vi "GSP_Manager_Wavelength_driver.vi"(4 "error in (no error)":errorcluster, 6 "Target (Move Only)":T1 {"Move type" items=["Both", "Grating Only", "Camera Only"]}, 7 "Action":T3) -> (0 "error out":errorcluster, 2 "VI reference (launch only)":refnum<vi>)   [LabVIEW 2015]
doc: "Provides an interface to the Camera Stage Manager. See the actions below.\n\nLaunch - launch the manager thread supplying references to the controls that the thread will update.\n\nHome - Home the camera stage\n\nMove - Move the camera to the position supplied by Target (in degrees)\n\nShutdown - Shutdown the camera stage manager"
uses:
  wavelength_driver_actions.ctl
  wavelength_parameters.ctl
  movetypes.ctl
  SystemUtil/Command.ctl
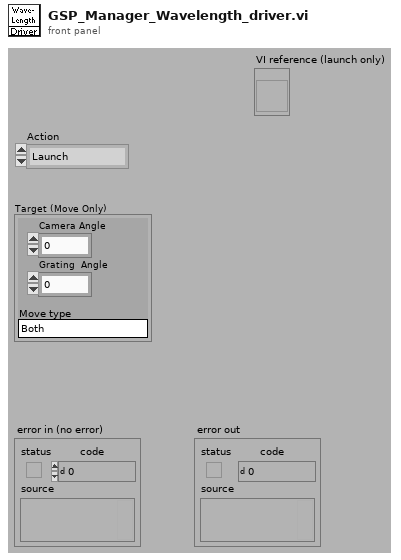
[diagram p1: front panel]
types:
  T1 = typedef "wavelength_parameters.ctl" = cluster{"Camera Angle":dbl, "Grating  Angle":dbl, "Move type":T2}
  T2 = typedef "movetypes.ctl" = u16
  T3 = typedef "wavelength_driver_actions.ctl" = enum16{"Launch", "Flexure On", "Flexure Off", "Move", "Home", "Shutdown"}
  T4 = typedef "Command.ctl" = cluster{"Command":string, "Parameter":string}
  T5 = cluster{string, "type string":i16[], "data string":string}
  T6 = cluster{string, "type string":i16[], "data string":string}[]
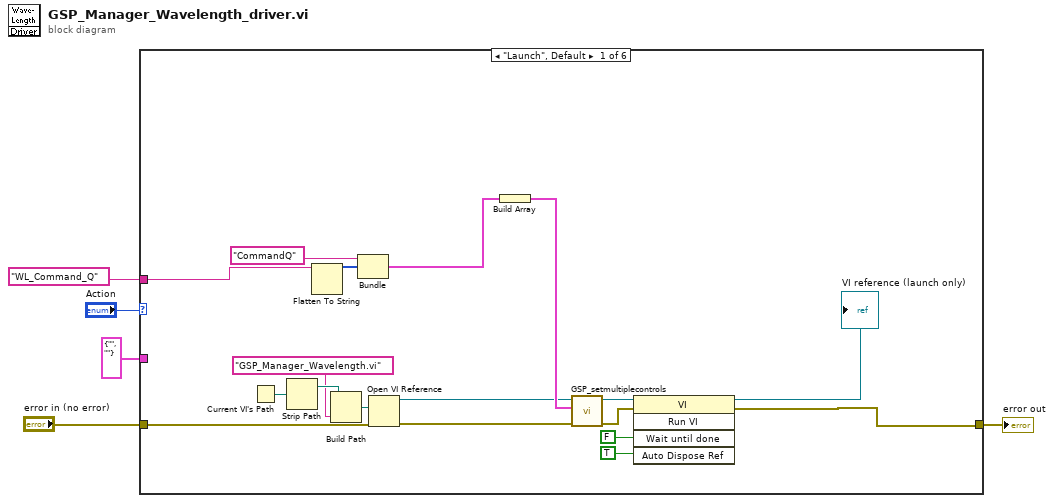
[diagram p0: block diagram]
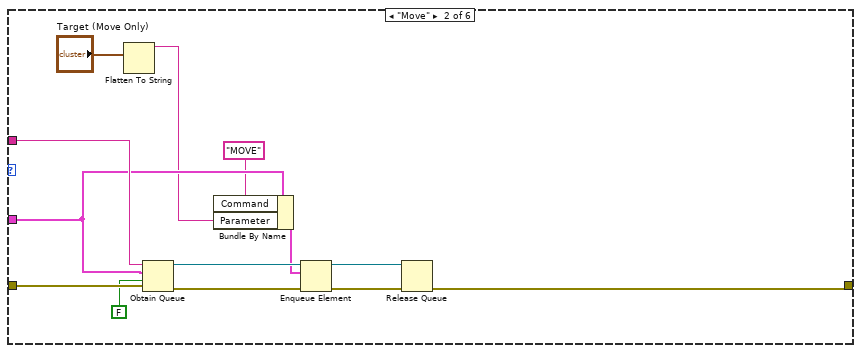
[diagram p2: hidden frame]
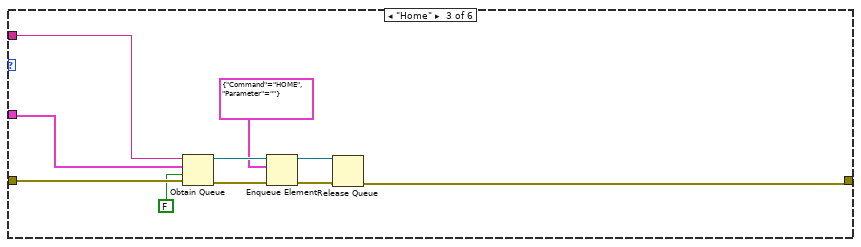
[diagram p3: hidden frame]
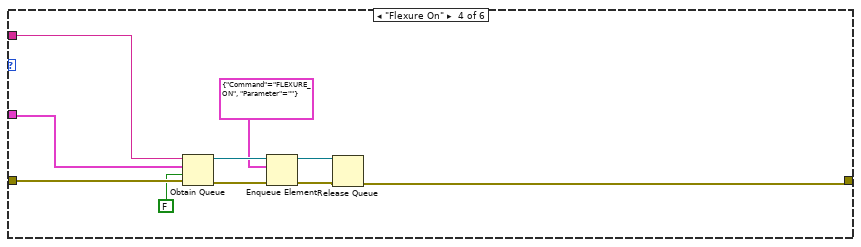
[diagram p4: hidden frame]
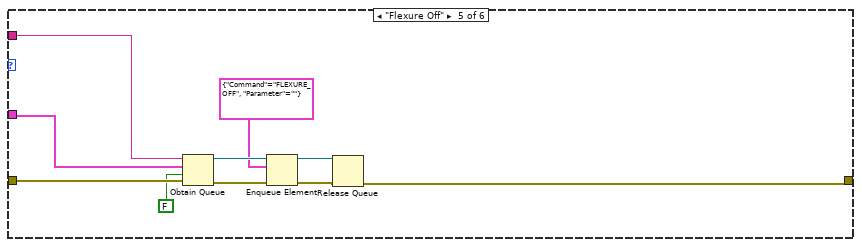
[diagram p5: hidden frame]
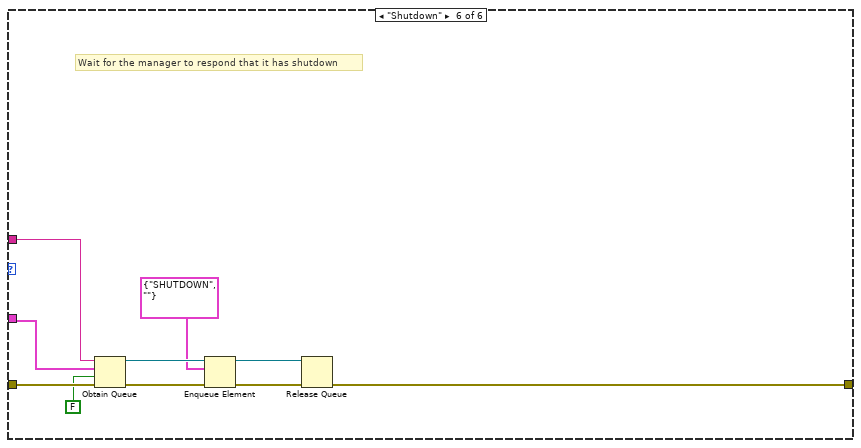
[diagram p6: hidden frame]
diagram:
  n1 = case shown="\"Launch\", Default" "Action" {
    tunnel: "error in (no error)" -> [w20 w37 w45 w55 w65 w77]
    tunnel: [w7 w25 w38 w48 w58 w68] -> w3
    tunnel: "WL_Command_Q" -> [w10 w35 w44 w54 w64 w74]
    tunnel: T4 {"Command"="", "Parameter"=""} ("Command") -> [_ w32 w42 w52 w62 w72]
    frame "Launch", Default {
      n2 = Current VI's Path() -> (path=w14:path)
      n3 = Strip Path(path=w14) -> (stripped path=w12:path)  [unwired: 1 out]
      n4 = Flatten To String(anything=w10) -> (data string=w22:string, type string=w23:i16[])  [unwired: 3 in, 1 out]
      n5 = Build Path(base path=w12, name or relative path="GSP_Manager_Wavelength.vi" ("vi path")) -> (appended path=w13:path)
      n6 = Bundle("CommandQ", "type string"=w23, "data string"=w22) -> (w8:T5)  [unwired: 1 in]
      n7 = Open VI Reference(vi path=w13, error in (no error)=w20) -> (vi reference=w9:refnum<vi>, error out=w19:errorcluster)  [unwired: 4 in]
      n8 = Build Array(w8) -> (w21:T6)
      n9 = call "GSP_setmultiplecontrols.vi"("error in (no error)"=w19, "Control Infos"=w21, "reference"=w9) -> ("error out"=w17:errorcluster, "reference out"=w18:refnum<vi>)  [unwired: 3 in]
      n10 = invoke class="VI" method="Run VI"(reference=w18, error in=w17, "Wait until done"=FALSE, "Auto Dispose Ref"=TRUE) -> (reference out=→"VI reference (launch only)":refnum<vi>, error out=w7:errorcluster)  [unwired: 1 in, 3 out]
    }
    frame "Move" {
      n11 = Flatten To String(anything="Target (Move Only)") -> (data string=w29:string)  [unwired: 3 in, 2 out]
      n12 = Obtain Queue(name (unnamed)=w35, element data type=w32, create if not found? (T)=FALSE, error in (no error)=w37) -> (queue out=w34:refnum<queue>, error out=w36:errorcluster)  [unwired: 1 in, 1 out]
      n13 = Bundle By Name(cluster=w32, "Command"="MOVE", "Parameter"=w29) -> (w31:T4)
      n14 = Enqueue Element(queue=w34, element=w31, error in (no error)=w36) -> (queue out=w27:refnum<queue>, error out=w26:errorcluster)  [unwired: 1 in, 1 out]
      n15 = Release Queue(queue=w27, error in (no error)=w26) -> (error out=w25:errorcluster)  [unwired: 1 in, 2 out]
    }
    frame "Home" {
      n16 = Obtain Queue(name (unnamed)=w44, element data type=w42, create if not found? (T)=FALSE, error in (no error)=w45) -> (queue out=w46:refnum<queue>, error out=w47:errorcluster)  [unwired: 1 in, 1 out]
      n17 = Enqueue Element(queue=w46, element=T4 {"Command"="HOME", "Parameter"=""}, error in (no error)=w47) -> (queue out=w40:refnum<queue>, error out=w39:errorcluster)  [unwired: 1 in, 1 out]
      n18 = Release Queue(queue=w40, error in (no error)=w39) -> (error out=w38:errorcluster)  [unwired: 1 in, 2 out]
    }
    frame "Flexure On" {
      n19 = Obtain Queue(name (unnamed)=w54, element data type=w52, create if not found? (T)=FALSE, error in (no error)=w55) -> (queue out=w56:refnum<queue>, error out=w57:errorcluster)  [unwired: 1 in, 1 out]
      n20 = Enqueue Element(queue=w56, element=T4 {"Command"="FLEXURE_ON", "Parameter"=""}, error in (no error)=w57) -> (queue out=w50:refnum<queue>, error out=w49:errorcluster)  [unwired: 1 in, 1 out]
      n21 = Release Queue(queue=w50, error in (no error)=w49) -> (error out=w48:errorcluster)  [unwired: 1 in, 2 out]
    }
    frame "Flexure Off" {
      n22 = Obtain Queue(name (unnamed)=w64, element data type=w62, create if not found? (T)=FALSE, error in (no error)=w65) -> (queue out=w66:refnum<queue>, error out=w67:errorcluster)  [unwired: 1 in, 1 out]
      n23 = Enqueue Element(queue=w66, element=T4 {"Command"="FLEXURE_OFF", "Parameter"=""}, error in (no error)=w67) -> (queue out=w60:refnum<queue>, error out=w59:errorcluster)  [unwired: 1 in, 1 out]
      n24 = Release Queue(queue=w60, error in (no error)=w59) -> (error out=w58:errorcluster)  [unwired: 1 in, 2 out]
    }
    frame "Shutdown" {
      # "Wait for the manager to respond that it has shutdown"
      n25 = Obtain Queue(name (unnamed)=w74, element data type=w72, create if not found? (T)=FALSE, error in (no error)=w77) -> (queue out=w75:refnum<queue>, error out=w76:errorcluster)  [unwired: 1 in, 1 out]
      n26 = Enqueue Element(queue=w75, element=T4 {"Command"="SHUTDOWN", "Parameter"=""}, error in (no error)=w76) -> (queue out=w70:refnum<queue>, error out=w69:errorcluster)  [unwired: 1 in, 1 out]
      n27 = Release Queue(queue=w70, error in (no error)=w69) -> (error out=w68:errorcluster)  [unwired: 1 in, 2 out]
    }
  }
  "error out" <- w3
